vi "niRFUtil WFM Detect Multiple Bursts.vi"   [LabVIEW 2015, in "niRFUtil.lvlib"]
uses:
  niRFUtil.lvlib
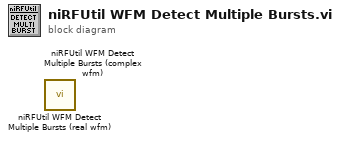
[diagram p0: block diagram]
diagram:
  n1 = call "niRFUtil WFM Detect Multiple Bursts (real wfm).vi"() -> ()  [unwired: 14 in, 2 out]
  n2 = call "niRFUtil WFM Detect Multiple Bursts (complex wfm).vi"() -> ()  [unwired: 14 in, 2 out]
